vi "Draw Matrix Plot.vi"(6 "Control Ref Queue":T4, 8 "error in (no error)":errorcluster, 10 "Matrix Representation Array In":T1, 11 "2D Plotmatrix.lvclass in":refnum<class "XY Plot Matrix.lvclass">) -> (0 "error out":errorcluster, 2 "Matrix Representation Array Out":T1, 3 "2D Plotmatrix.lvclass out":refnum<class "XY Plot Matrix.lvclass">)   [LabVIEW 2020, in "XY Plot Matrix.lvclass"]
uses:
  <vilib>/Math Plots/2D Math Plots/XY Plot Matrix/XY Plot Matrix/XY Plot Matrix.lvclass
  <vilib>/Math Plots/2D Math Plots/XY Plot Matrix/XY Plot Matrix/Typedef/Mulitmatrix Representation.ctl
  <vilib>/Math Plots/2D Math Plots/XY Plot Matrix/XY Plot Matrix/Typedef/Matrix Representation.ctl
  <vilib>/Math Plots/2D Math Plots/2D Plot/2D Plot/Typedef/Range Cluster.ctl
  <vilib>/Math Plots/2D Math Plots/2D Plot/Action String/XYPlotMatrix Ctrl Act Queue.ctl
  <vilib>/Math Plots/2D Math Plots/2D Plot/Action String/XYPlotMatrix Ctrl Act Cluster.ctl
  <vilib>/Math Plots/2D Math Plots/2D Plot/Action String/2DMathPlot State Class.ctl
  e:/builds/penguin/labview/branches/2020/dev/dist/vi.lib/Math Plots/2D Math Plots/2D Plot/2D Plot/2D Plot.lvclass
  <vilib>/Math Plots/2D Math Plots/XY Plot Matrix/XY Plot Matrix/XY Plot Matrix.lvclass/XY Plot Matrix.ctl
  <vilib>/Math Plots/2D Math Plots/2D Plot/2D Plot/2D Plot.lvclass
  <vilib>/Math Plots/Plot Private Lib/NI_Math Plot Private Lib.lvlib
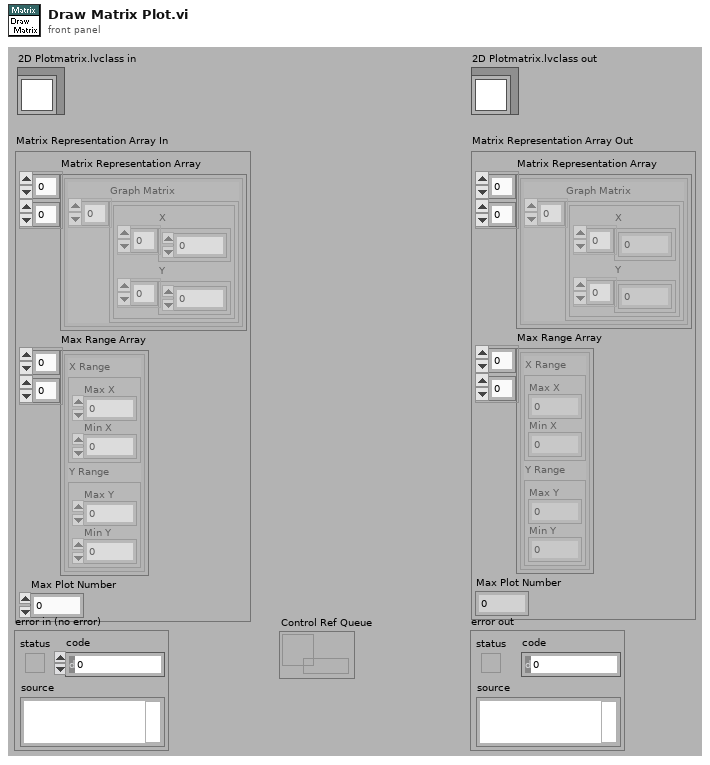
[diagram p1: front panel]
types:
  T1 = typedef "XY Plot Matrix.lvclass/Mulitmatrix Representation.ctl" = cluster{"Matrix Representation Array":T2[][], "Max Range Array":T3[][], "Max Plot Number":i32}
  T2 = typedef "XY Plot Matrix.lvclass/Matrix Representation.ctl" = cluster{"Graph Matrix":cluster{"X":dbl[], "Y":dbl[]}[]}
  T3 = typedef "2D Plot.lvclass/Range Cluster.ctl" = cluster{"X Range":cluster{"Max X":dbl, "Min X":dbl}, "Y Range":cluster{"Max Y":dbl, "Min Y":dbl}}
  T4 = typedef "XYPlotMatrix Ctrl Act Queue.ctl" = refnum<queue>
  T5 = typedef "2DMathPlot State Class.ctl" = enum16{"Update All (Undo)", "Update General", "Update Appearance", "Update Format", "Update Scale", "Update Marker", "Update Cursor", "None"}
  T6 = typedef "XY Plot Matrix.lvclass/Plotmatrix Property Array.ctl" = T7[][]
  T7 = typedef "XY Plot Matrix.lvclass/Plotmatrix Property.ctl" = cluster{"Plot Property Array":T8}
  T8 = typedef "2D Plot.lvclass/Plot Property Array.ctl" = T9[]
  T9 = typedef "2D Plot.lvclass/Plot Property.ctl" = cluster{"Bar Plot Style":u8, "DigitalLineStyle":u8, "TransitionLocation":u8, "Transition Type":u8, "Fill To":i16, "Fill/Pt. Color":u32, "Label Style":u8, "Line Style":u8, "Line Width":u8, "Plot Color":u32, "Plot Interpolation":u8, "Plot Name":string, "Point Style":u8, "Visible?":bool, "XScaleIdx":u32, "YScaleIdx":u32}
  T10 = typedef "XYPlotMatrix Ctrl Act Cluster.ctl" = cluster{"Facade VI":refnum<vi>, "XControl":refnum<vi>, "Sub Panel":refnum<vi>, "Sub VI":refnum<vi>, "Export Image":refnum<vi>, "Display State Change Class":T5}
  T11 = typedef "2D Plot.lvclass/Property Cluster.ctl" = cluster{"Graph General":T12, "Format Property":string[], "Scale Array":T13, "Cursor Property":T16, "Annotation List":T18, "Active Cursor":i32, "Active Plot":i32}
  T12 = typedef "2D Plot.lvclass/Graph General Property.ctl" = cluster{"Palette Visible":cluster{"Graph Legend":bool, "Plot Legend":bool, "Auto size":bool, "Number of Plots":u32, "X Scrollbar":bool, "Scale Legend":bool, "Cursor Legend":bool}, "Plot Area Color":cluster{"FG Color":u32, "BG Color":u32}, "Bounds Size":cluster{"Width":u32, "Height":u32}, "Plot Area Bounds":cluster{"Left":i16, "Top":i16, "Right":i16, "Bottom":i16}}
  T13 = typedef "2D Plot.lvclass/Scale Array.ctl" = T14[]
  T14 = typedef "2D Plot.lvclass/Scale Cluster.ctl" = cluster{"General":cluster{"Editable":bool, "Flipped":bool, "Mapping Mode":u8, "Visible":bool, "Style":u8, "Scale Fit":u8}, "Offset and Multiplier":T15, "Range":cluster{"Minimum":dbl, "Maximum":dbl, "Increment":dbl, "Minor Increment":dbl, "Start":dbl}, "Tick Color":cluster{"Major Color":u32, "Minor Color":u32}, "Gird Color":cluster{"Major Color":u32, "Minor Color":u32}, "Marker":cluster{"Visible":bool, "FG Color":u32, "BG Color":u32, "Font Name":string, "Font Size":u32, "Font Bold":bool, "Font Italic":bool, "Font Strikeout":bool, "Font Underline":bool}, "Name Label":cluster{"Visible":bool, "FG Color":u32, "BG Color":u32, "Font Name":string, "Font Size":u32, "Font Bold":bool, "Font Italic":bool, "Font Strikeout":bool, "Font Underline":bool, "Justification":enum16{"Left", "Center", "Right"}, "Text":string}}
  T15 = typedef "LVOffsetAndMultiplierTypeDef.ctl" = cluster{"Offset":dbl, "Multiplier":dbl}
  T16 = typedef "2D Plot.lvclass/Cursor Property.ctl" = cluster{"Cursor List":T17, "Cursor List Addtional":cluster{"Cursor Selection Color":u32, "Line Style":u8, "Line Width":u8, "Visible":bool}[]}
  T17 = typedef "LVCursorListTypeDef.ctl" = cluster{"Name":string, "Color":u32, "Style":u8, "Point Style":u8, "Name Visible":bool, "Allow Drag":bool, "Cursor Mode":u32, "Plot":i32, "Index":i32, "Position":cluster{"X":dbl, "Y":dbl}, "X Scale":u32, "Y Scale":u32, "Watch Plots":i32[], "Watch All Plots":bool, "Plot Area":i32, "Label Offset":cluster{"X":dbl, "Y":dbl}}[]
  T18 = typedef "LVAnnotationListTypeDef.ctl" = cluster{"Name":string, "Color":u32, "Style":u8, "Point Style":u8, "Name Visible":bool, "Allow Drag":bool, "Annotation Mode":u32, "Plot":i32, "Index":i32, "Position":cluster{"X":dbl, "Y":dbl}, "X Scale":u32, "Y Scale":u32, "Show Arrow":bool, "Lock Name":bool, "Plot Area":i32, "Label Offset":cluster{"X":dbl, "Y":dbl}}[]
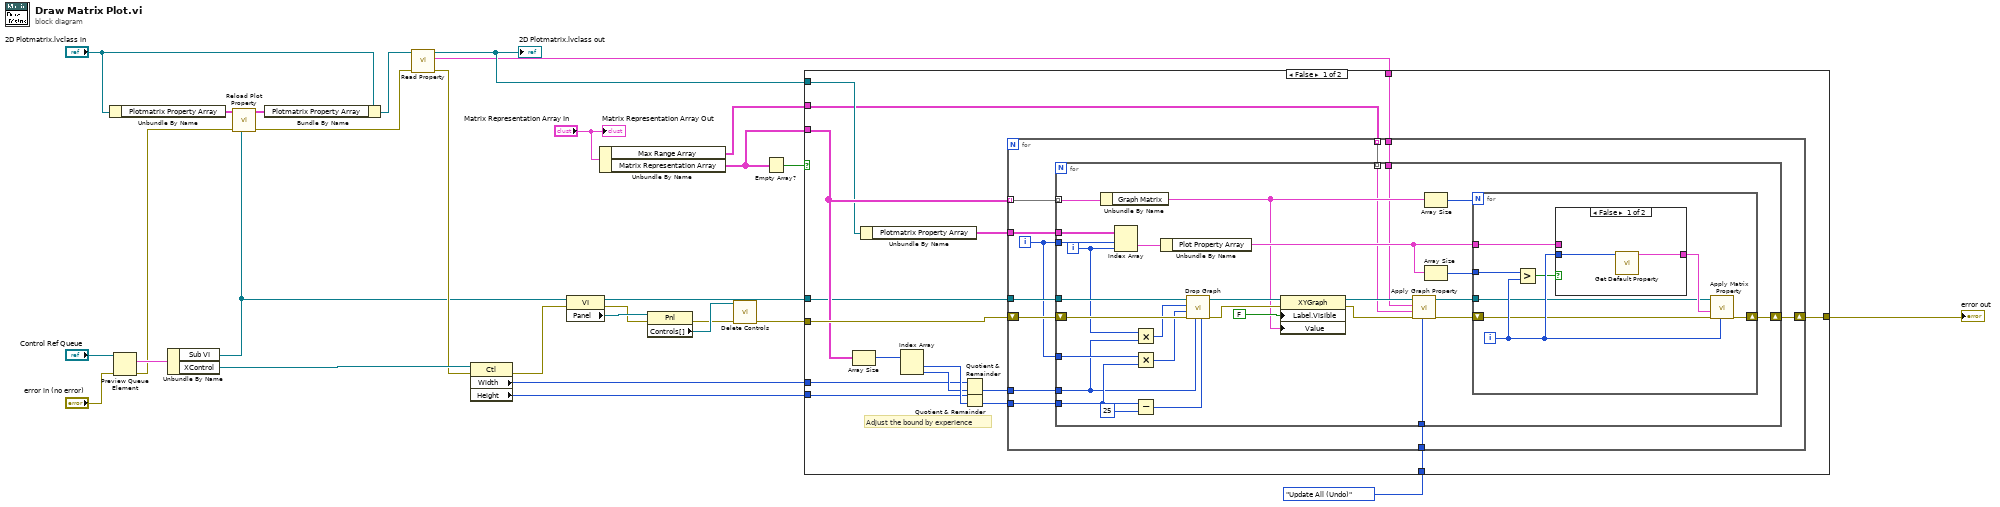
[diagram p0: block diagram]
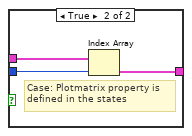
[diagram p2: hidden frame]
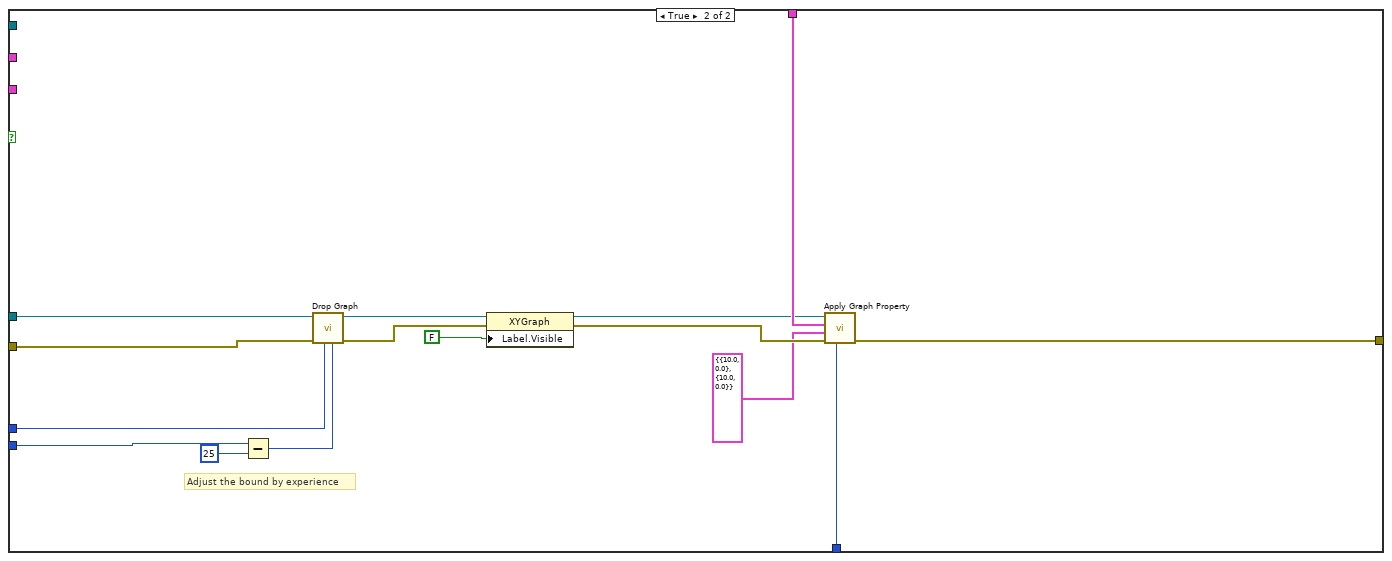
[diagram p3: hidden frame]
diagram:
  n1 = Unbundle By Name("2D Plotmatrix.lvclass in") -> ("Plotmatrix Property Array"=w7:T6)
  n2 = Preview Queue Element(queue="Control Ref Queue", error in (no error)="error in (no error)") -> (element=w28:T10, error out=w3:errorcluster)  [unwired: 3 out]
  n3 = Unbundle By Name(w28) -> ("Sub VI"=w4:refnum<vi>, "XControl"=w26:refnum<vi>)
  n4 = call <vilib>:"Reload Plot Property.vi"("Sub VI"=w4, "error in (no error)"=w3, "Plot Property Array In"=w7) -> ("error out"=w2:errorcluster, "Plot Property Array Out"=w8:T6)  [unwired: 7 out]
  n5 = Bundle By Name(cluster="2D Plotmatrix.lvclass in", "Plotmatrix Property Array"=w8) -> (w5:refnum<class "XY Plot Matrix.lvclass">)
  n6 = call <vilib>:"Read Property.vi"("error in (no error)"=w2, "2D Plot.lvclass in"=w5) -> ("error out"=w13:errorcluster, "XY Graph Property Cluster"=w9:T11, "2D Plot.lvclass out"=w14:refnum<class "XY Plot Matrix.lvclass">)  [unwired: 7 out]
  "2D Plotmatrix.lvclass out" <- w14
  n7 = property class="Ctl"(reference=w26, error in=w13) -> (error out=w21:errorcluster, "Width"=w12:u32, "Height"=w16:u32)  [unwired: 1 out]
  n8 = property class="VI"(reference=w4, error in=w21) -> (reference out=w20:refnum<vi>, error out=w24:errorcluster, "Panel"=w25:refnum<vi>)
  n9 = Unbundle By Name("Matrix Representation Array In") -> ("Max Range Array"=w10:T3[][], "Matrix Representation Array"=w15:T2[][])
  n10 = property class="Pnl"(reference=w25, error in=w24) -> (error out=w18:errorcluster, "Controls[]"=w23:refnum<vi>[])  [unwired: 1 out]
  n11 = call <vilib>:"Delete Controls.vi"("error in (no error)"=w18, "Controls[]"=w23) -> ("error out"=w22:errorcluster)  [unwired: 9 out]
  n12 = Empty Array?(array=w15) -> (empty?=w17:bool)
  n13 = case shown="False" w17 {
    tunnel: w22 -> [w45 w102]
    tunnel: w12 -> [w31 w100]
    tunnel: w16 -> [w30 w112]
    tunnel: w14 -> [w35 _]
    tunnel: w20 -> [w37 w104]
    tunnel: [w36 w109] -> w1
    tunnel: w15 -> [w39 _]
    tunnel: w9 -> [w34 w108]
    tunnel: 2DMathPlot_State_Class."Update All (Undo)" ("Display State Change Class") -> [w33 w106]
    tunnel: w10 -> [w32 _]
    frame False {
      # "Adjust the bound by experience"
      n14 = Array Size(array=w39) -> (size(s)=w42:i32[])
      n15 = Unbundle By Name(w35) -> ("Plotmatrix Property Array"=w38:T6)
      n16 = Index Array(array=w42) -> (element #1=w41:i32, element #2=w40:i32)  [unwired: 2 in]
      n17 = Quotient & Remainder(x=w31, y=w40) -> (floor(x/y)=w43:u32)  [unwired: 1 out]
      n18 = Quotient & Remainder(x=w30, y=w41) -> (floor(x/y)=w44:u32)  [unwired: 1 out]
      n19 = for {
        tunnel: w37 -> [w56]
        shift-right: [w55] -> w36
        shift-left: w45 -> [w54]
        tunnel: w44 -> [w53]
        tunnel: w43 -> [w52]
        tunnel: w39 -> [w51] mode=indexing
        tunnel: w38 -> [w49]
        tunnel: w34 -> [w50]
        tunnel: w33 -> [w47]
        tunnel: w32 -> [w46] mode=indexing
        i -> [w48]
        n20 = for {
          tunnel: w56 -> [w85]
          tunnel: w48 -> [w84]
          shift-right: [w74] -> w55
          shift-left: w54 -> [w83]
          tunnel: w53 -> [w82]
          tunnel: w52 -> [w57]
          tunnel: w51 -> [w77] mode=indexing
          tunnel: w49 -> [w76]
          tunnel: w50 -> [w65]
          tunnel: w48 -> [w64]
          tunnel: w47 -> [w62]
          tunnel: w46 -> [w61] mode=indexing
          i -> [w63]
          n21 = Unbundle By Name(w77) -> ("Graph Matrix"=w71:cluster{"X":dbl[], "Y":dbl[]}[])
          n22 = Index Array(array=w76, index (row)=w64, index (col)=w63) -> (element=w75:T7)
          n23 = Multiply(x=w63, y=w57) -> (x*y=w59:u32)
          n24 = Multiply(x=w84, y=w82) -> (x*y=w58:u32)
          n25 = Subtract(x=w82, y=u32 25) -> (x-y=w60:u32)
          n26 = Unbundle By Name(w75) -> ("Plot Property Array"=w73:T8)
          n27 = call <vilib>:"Drop Graph.vi"("Height"=w60, "Width"=w57, "error in (no error)"=w83, "Vertical"=w58, "Horizontal"=w59, "Sub VI"=w85) -> ("error out"=w79:errorcluster, "XY Graph ref"=w81:refnum<vi>)  [unwired: 4 out]
          n28 = property class="XYGraph"(reference=w81, error in=w79, "Label.Visible"=FALSE, "Value"=w71) -> (reference out=w69:refnum<vi>, error out=w67:errorcluster)
          n29 = call <vilib>:"Apply Graph Property.vi"("Display State Change Class"=w62, "error in (no error)"=w67, "Max Range"=w61, "XY Graph Property Cluster"=w65, "XY Graph"=w69) -> ("error out"=w66:errorcluster, "XY Graph"=w68:refnum<vi>)  [unwired: 2 in, 3 out]
          n30 = Array Size(array=w71) -> (size(s)=w70:i32)
          n31 = Array Size(array=w73) -> (size(s)=w72:i32)
          n32 = for {
            N: w70 -> [_]
            tunnel: w73 -> [w92]
            tunnel: w68 -> [w86]
            shift-right: [w91] -> w74
            shift-left: w66 -> [w87]
            tunnel: w72 -> [w90]
            i -> [w89]
            n33 = Greater?(x=w90, y=w89) -> (0:w88:bool)
            n34 = case shown="False" w88 {
              tunnel: w92 -> [_ w98]
              tunnel: w89 -> [w95 w97]
              tunnel: [w94 w96] -> w93
              frame False {
                n35 = call <vilib>:"Get Default Property.vi"("Index"=w95) -> ("Temporary Property"=w94:T9)  [unwired: 3 in, 7 out]
              }
              frame True {
                # "Case: Plotmatrix property is \ndefined in the states"
                n36 = Index Array(array=w98, index=w97) -> (element=w96:T9)
              }
            }
            n37 = call <vilib>:"Apply Matrix Property.vi"("Plot ID"=w89, "error in (no error)"=w87, "Plot Property"=w93, "Polar Area Ref In"=w86) -> ("error out"=w91:errorcluster)  [unwired: 1 in, 6 out]
          }
        }
      }
    }
    frame True {
      # "Adjust the bound by experience"
      n38 = Subtract(x=w112, y=u32 25) -> (x-y=w99:u32)
      n39 = call <vilib>:"Drop Graph.vi"("Height"=w99, "Width"=w100, "error in (no error)"=w102, "Sub VI"=w104) -> ("error out"=w101:errorcluster, "XY Graph ref"=w103:refnum<vi>)  [unwired: 2 in, 4 out]
      n40 = property class="XYGraph"(reference=w103, error in=w101, "Label.Visible"=FALSE) -> (reference out=w107:refnum<vi>, error out=w110:errorcluster)
      n41 = call <vilib>:"Apply Graph Property.vi"("Display State Change Class"=w106, "error in (no error)"=w110, "Max Range"=T3 {"X Range"={"Max X"=10.0, "Min X"=0.0}, "Y Range"={"Max Y"=10.0, "Min Y"=0.0}}, "XY Graph Property Cluster"=w108, "XY Graph"=w107) -> ("error out"=w109:errorcluster)  [unwired: 1 in, 5 out]
    }
  }
  "error out" <- w1
  "Matrix Representation Array Out" <- "Matrix Representation Array In"
